vi "Handle Last Ack Core.vi"(4 "error in (no error)":errorcluster, 6 "Last Ack":refnum<class "Last Ack.lvclass">, 7 "Camera Display in":refnum<class "Camera Display.lvclass">) -> (0 "error out":errorcluster, 3 "Camera Display out":refnum<class "Camera Display.lvclass">)   [LabVIEW 2014, in "Camera Display.lvlib" / "Camera Display.lvclass"]
doc: "(<B>Filename</B>: Actor Framework.lvlib:Actor.lvclass:Handle Last Ack Core.vi)\n\nDefines how the caller actor responds to the Last Ack message from a nested actor. The Last Ack message is the final message a nested actor sends to its caller before it shuts down. The message contains information about the final state of the nested actor.\n\nBy default, this method does nothing except return any error the nested actor sent. A descendant class may override this method to define behavior."
uses:
  Camera Display.lvclass
  <vilib>/ActorFramework/LastAck/Last Ack.lvclass
  Camera Dir Dialog/Camera Dir Dialog/Camera Dir Dialog.lvclass
  <vilib>/ActorFramework/LastAck/Last Ack.lvclass/Last Ack.ctl
  Camera Dir Dialog/Camera Dir Dialog/Camera Dir Dialog.lvclass/Camera Dir Dialog.ctl
  Camera Display.lvclass/Camera Display.ctl
  Camera Dir Dialog/Camera Dir Dialog/Read Config Dir.vi
  Camera Dir Dialog/Camera Dir Dialog/Read WorkDir.vi
  Shared Code/Viewable Actor/ViewableActor/ViewableActor.lvclass
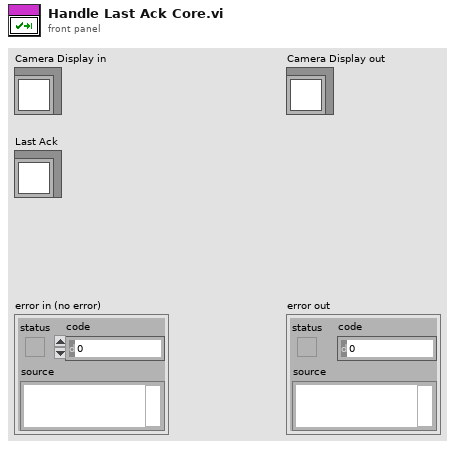
[diagram p1: front panel]
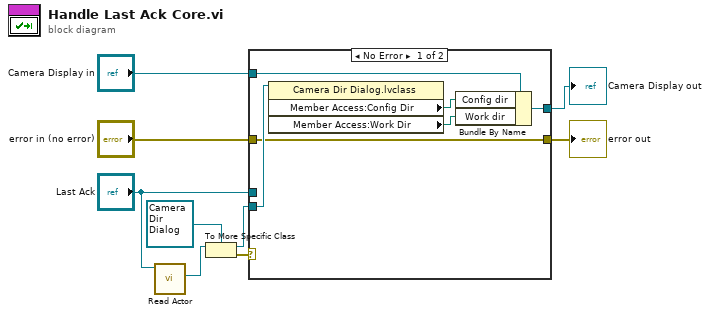
[diagram p0: block diagram]
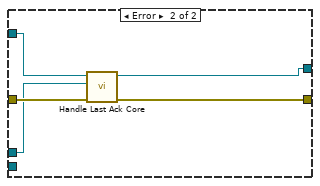
[diagram p2: hidden frame]
diagram:
  n1 = call <vilib>:"Read Actor.vi"("Last Ack"="Last Ack") -> ("Actor"=w9:refnum<class "Actor.lvclass">)  [unwired: 10 in]
  n2 = To More Specific Class(target class=refnum<class "Camera Dir Dialog.lvclass"> refnum ("Camera Dir Dialog.lvlib:Camera Dir Dialog.lvclass"), reference=w9) -> (specific class reference=w6:refnum<class "Camera Dir Dialog.lvclass">, error out=w5:errorcluster)  [unwired: 1 in]
  n3 = case shown="No Error" w5 {
    tunnel: "Camera Display in" -> [w15 w20]
    tunnel: [w14 w19] -> w7
    tunnel: w6 -> [w13 _]
    tunnel: "error in (no error)" -> [w10 w18]
    tunnel: [w10 w17] -> w2
    tunnel: "Last Ack" -> [_ w16]
    frame No Error {
      n4 = property class="Camera Dir Dialog.lvclass"(reference=w13) -> ("Member Access:Config Dir"=w12:path, "Member Access:Work Dir"=w11:path)  [unwired: 1 in, 2 out]
      n5 = Bundle By Name(cluster=w15, "Config dir"=w12, "Work dir"=w11) -> (w14:refnum<class "Camera Display.lvclass">)
    }
    frame Error {
      n6 = call-parent "Handle Last Ack Core.vi"("error in (no error)"=w18, "Last Ack"=w16, "Actor in"=w20) -> ("error out"=w17:errorcluster, "Actor out"=w19:refnum<class "Camera Display.lvclass">)  [unwired: 3 in]
    }
  }
  "Camera Display out" <- w7
  "error out" <- w2
